vi "Read Analogue.vi"(8 "error in (no error)":errorcluster, 11 "Chroma190020 HiPOT in":refnum<class "Chroma190020 HiPOT.lvclass">) -> (0 "error out":errorcluster, 2 "Measurements":dbl, 3 "Chroma190020 HiPOT out":refnum<class "Chroma190020 HiPOT.lvclass">)   [LabVIEW 2021, in "Concrete.lvlib" / "Chroma190020 HiPOT.lvclass"]
uses:
  Chroma190020 HiPOT.lvclass
  Chroma190020 HiPOT.lvclass/Chroma190020 HiPOT.ctl
  Harware Abstraction/AnalogIO/AIO.lvclass
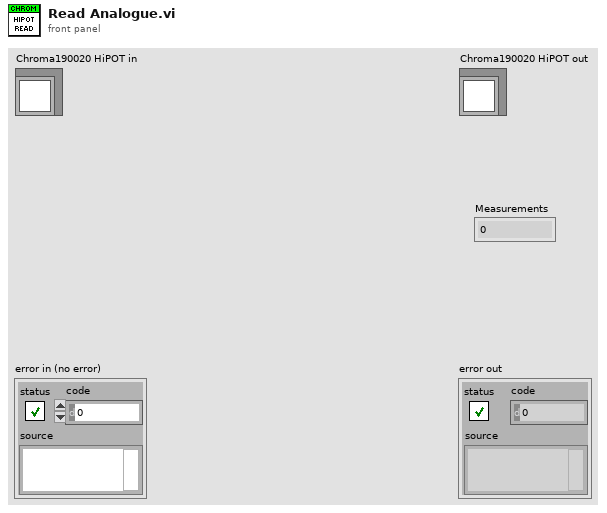
[diagram p1: front panel]
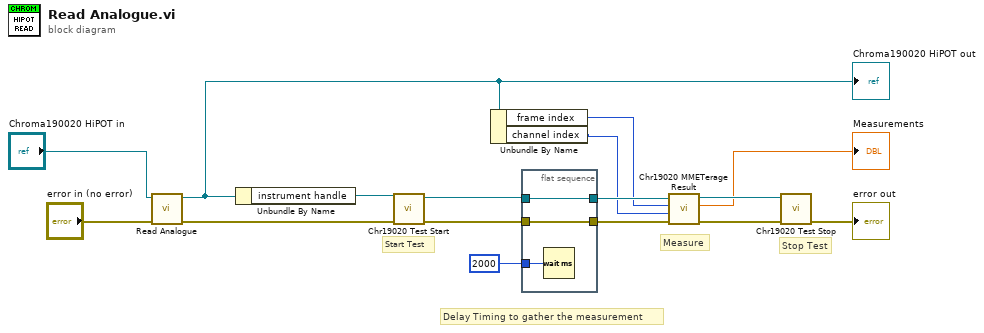
[diagram p0: block diagram]
diagram:
  # "Delay Timing to gather the measurement"
  # "Stop Test"
  # "Start Test"
  # "Measure"
  n1 = call-parent "Read Analogue.vi"("error in (no error)"="error in (no error)", "PS in"="Chroma190020 HiPOT in") -> ("error out"=w10:errorcluster, "PS out"=w3:refnum<class "Chroma190020 HiPOT.lvclass">)  [unwired: 7 in, 1 out]
  "Chroma190020 HiPOT out" <- w3
  n2 = Unbundle By Name(w3) -> ("instrument handle"=w9:refnum<k15>)
  n3 = call <instrlib>:"Chr19020 Test Start.vi"("error in (no error)"=w10, "instrument handle"=w9) -> ("error out"=w8:errorcluster, "instrument handle out"=w6:refnum<k15>)  [unwired: 8 in]
  n4 = Unbundle By Name(w3) -> ("frame index"=w2:i32, "channel index"=w1:i32)
  n5 = flat-sequence {
    tunnel: u32 2000 -> [w17]
    tunnel: [w19] -> w7
    tunnel: w8 -> [w19]
    tunnel: [w18] -> w5
    tunnel: w6 -> [w18]
    frame #0 {
      n6 = Wait (ms)(milliseconds to wait=w17) -> ()  [unwired: 1 out]
    }
  }
  n7 = call <instrlib>:"Chr19020 MMETerage Result.vi"("error in (no error)"=w7, "channel index"=w1, "frame index"=w2, "instrument handle"=w5) -> ("error out"=w14:errorcluster, "return value"=→"Measurements":dbl, "instrument handle out"=w13:refnum<k15>)  [unwired: 5 in]
  n8 = call <instrlib>:"Chr19020 Test Stop.vi"("error in (no error)"=w14, "instrument handle"=w13) -> ("error out"=→"error out":errorcluster)  [unwired: 8 in, 1 out]
